vi "Error Write Watch.vi"(8 "error in":errorcluster, 10 "Watchdog STS":i32, 11 "Error in":refnum<class "Error.lvclass">) -> (0 "error out":errorcluster, 3 "Error out":refnum<class "Error.lvclass">)   [LabVIEW 2023, in "Error.lvclass"]
uses:
  Error.lvclass
  <vilib>/ADAS Replay HIL/Channels/Tag Wrapper/Tag Wrapper.lvlib
  <vilib>/ADAS Replay HIL/Channels/Tag Wrapper/Polymorphic/Write Channel (I32).vi
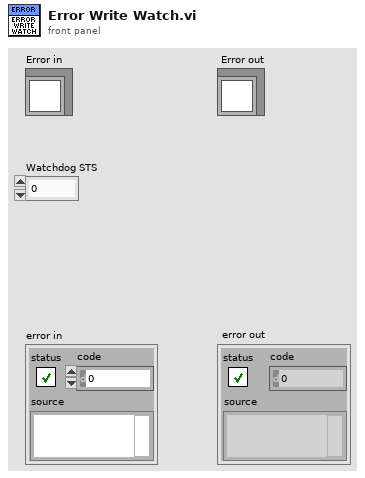
[diagram p1: front panel]
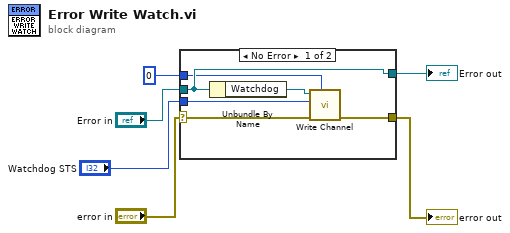
[diagram p0: block diagram]
diagram:
  n1 = case shown="No Error" "error in" {
    selector: "error in" -> [w12 w14]
    tunnel: [w11 w14] -> w5
    tunnel: "Error in" -> [w9 w13]
    tunnel: [w9 w13] -> w2
    tunnel: "Watchdog STS" -> [w10 _]
    tunnel: 0 ("Timeout (ms)") -> [w7 _]
    frame No Error {
      n2 = Unbundle By Name(w9) -> ("Watchdog"=w8:refnum<k21>)
      n3 = call-poly <vilib>:"Write Channel.vi"("Timeout (ms)"=w7, "error in"=w12, "Value to Write"=w10, "ADAS HIL Channel in"=w8) -> ("error out"=w11:errorcluster)  [unwired: 5 in, 2 out]
    }
    frame Error {
    }
  }
  "error out" <- w5
  "Error out" <- w2
